vi "sub vi - check network dir v2.vi"(11 "PATH":path) -> (0 "error":bool)   [LabVIEW 2017]
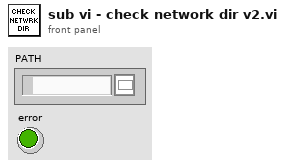
[diagram p1: front panel]
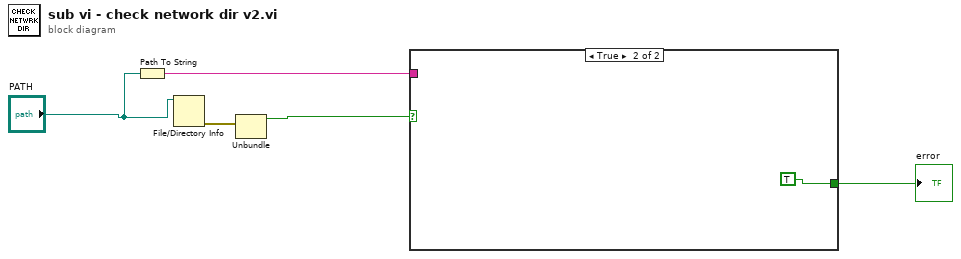
[diagram p0: block diagram]
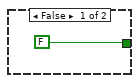
[diagram p2: hidden frame]
diagram:
  n1 = Path To String(path="PATH") -> (string=w5:string)
  n2 = File/Directory Info(path="PATH") -> (error out=w3:errorcluster)  [unwired: 1 in, 6 out]
  n3 = Unbundle(w3) -> ("status"=w4:bool)  [unwired: 2 out]
  n4 = case shown="True" w4 {
    tunnel: w5 -> [_ _]
    tunnel: [FALSE TRUE] -> w2
    frame False {
    }
    frame True {
    }
  }
  "error" <- w2
